vi "Popup Dialog CLBK.vi"(6 "show":bool, 8 "error in":errorcluster, 9 "String":string, 10 "Delay (5sec)":dbl, 11 "Tab Control":T1) -> (0 "error out":errorcluster, 2 "canceled?":bool, 3 "Answer MSG":string)   [LabVIEW 2020, in "Popup Dialog.lvlib"]
uses:
  Popup Dialog.lvlib
  Popup Dialog States.ctl
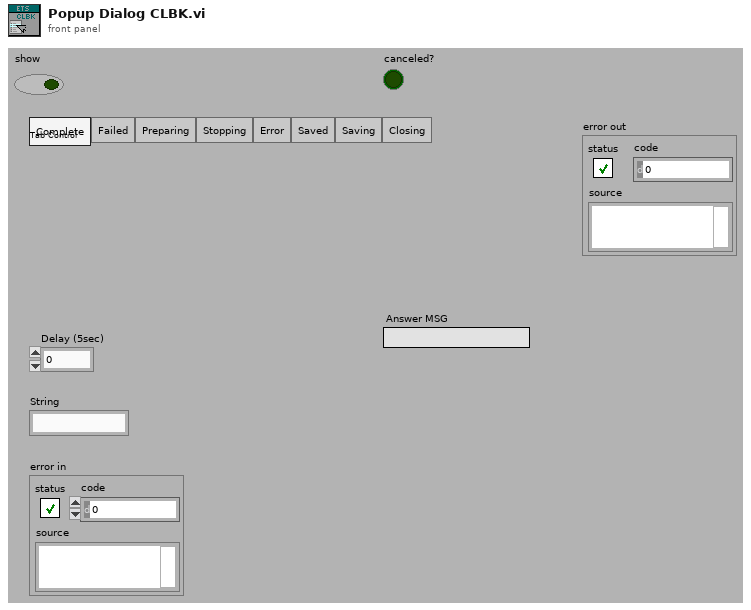
[diagram p1: front panel]
types:
  T1 = typedef "Popup Dialog.lvlib/Popup Dialog States.ctl" = enum32{"Complete", "Failed", "Preparing", "Stopping", "Error", "Saved", "Saving", "Closing"}
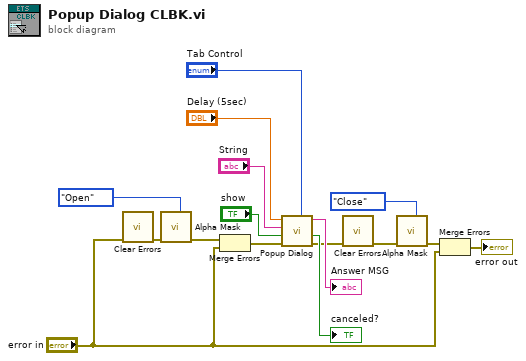
[diagram p0: block diagram]
diagram:
  n1 = call <vilib>:"Clear Errors.vi"("error in (no error)"="error in") -> ("error out"=w1:errorcluster)  [unwired: 5 in, 1 out]
  n2 = call "Alpha Mask.vi"("State"=enum16{"Init", "Open", "Close"}."Open", "error in (no error)"=w1) -> ("error out"=w7:errorcluster)  [unwired: 8 in, 1 out]
  n3 = Merge Errors(w7, "error in") -> (w8:errorcluster)
  n4 = call "Popup Dialog.vi"("Tab Control"="Tab Control", "error in (no error)"=w8, "show"="show", "Error MSG"="String", "Delay (5sec)"="Delay (5sec)") -> ("error out"=w5:errorcluster, "canceled?"=→"canceled?":bool, "Answer MSG"=→"Answer MSG":string)  [unwired: 4 in]
  n5 = call <vilib>:"Clear Errors.vi"("error in (no error)"=w5) -> ("error out"=w4:errorcluster)  [unwired: 5 in, 1 out]
  n6 = call "Alpha Mask.vi"("State"=enum16{"Init", "Open", "Close"}."Close", "error in (no error)"=w4) -> ("error out"=w3:errorcluster)  [unwired: 8 in, 1 out]
  n7 = Merge Errors(w3, "error in") -> (→"error out":errorcluster)
